vi "Gear Mech Global.vi"() -> ()   [LabVIEW 2016]
panel:
  in  "Full Up Position":dbl=600.0
  in  "Down Position":dbl=345.0
  in  "Up Position":dbl=560.0
  in  "In Speed":dbl=0.5
  in  "Out Speed":dbl=-0.5
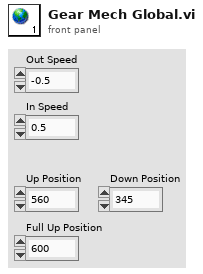
[diagram p1: front panel]
diagram:
